vi "SPCM test run.vi"() -> ()   [LabVIEW 2025]
uses:
  <vilib>/DAQmx/create/channels.llb/DAQmx Create Channel (CI-Count Edges).vi
  <vilib>/DAQmx/miscellaneous.llb/DAQmx Fill In Error Info.vi
  <vilib>/DAQmx/read.llb/DAQmx Read (Counter U32 1Chan 1Samp).vi
panel:
  out "data":u32
  out "Time has Elapsed":bool
  in  "Counter path":string
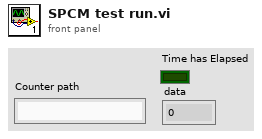
[diagram p1: front panel]
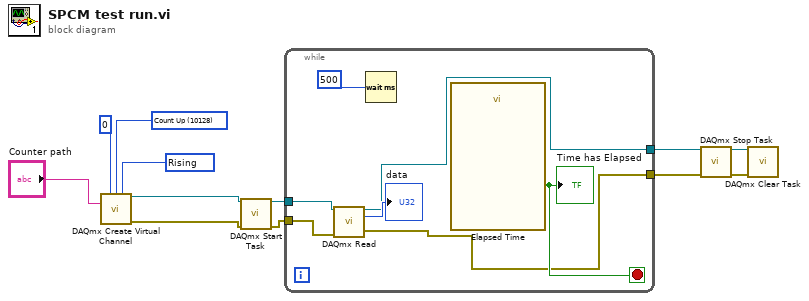
[diagram p0: block diagram]
diagram:
  w9 = 10280 items=["Rising"=10280, "Falling"=10171] ("edge")
  w10 = 10128 items=["Count Up"=10128, "Count Down"=10124, "Externally Controlled"=10326] ("count direction")
  n1 = call-poly <vilib>:"DAQmx Create Virtual Channel.vi"("initial count"=u32 0, "count direction"=w10, "edge"=w9, "counter"="Counter path") -> ("task out"=w8:refnum<k21>, "error out"=w6:errorcluster)  [unwired: 10 in]
  n2 = call <vilib>:"DAQmx Start Task.vi"("task/channels in"=w8, "error in"=w6) -> ("task out"=w7:refnum<k21>, "error out"=w3:errorcluster)  [unwired: 12 in]
  n3 = while {
    tunnel: w7 -> [w19]
    tunnel: w3 -> [w14]
    tunnel: [w13] -> w2
    tunnel: [w15] -> w1
    stop <- w17 stop-if-true
    n4 = call-poly <vilib>:"DAQmx Read.vi"("task/channels in"=w19, "error in"=w14) -> ("task out"=w15:refnum<k21>, "data"=→"data":u32, "error out"=w13:errorcluster)  [unwired: 11 in]
    n5 = Wait (ms)(milliseconds to wait=u32 500) -> ()  [unwired: 1 out]
    n6 = call "Elapsed Time"() -> ("Time has Elapsed"=w17:bool)  [unwired: 12 in, 7 out]
    "Time has Elapsed" <- w17
  }
  n7 = call <vilib>:"DAQmx Stop Task.vi"("task/channels in"=w1, "error in"=w2) -> ("task out"=w5:refnum<k21>, "error out"=w4:errorcluster)  [unwired: 12 in]
  n8 = call <vilib>:"DAQmx Clear Task.vi"("task in"=w5, "error in"=w4) -> ()  [unwired: 13 in, 1 out]
